vi "Main.vi"() -> ()   [LabVIEW 2015]
panel:
  out "data value":i32[][](array[numeric])
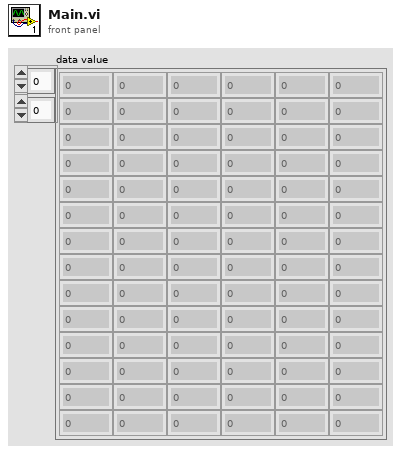
[diagram p1: front panel]
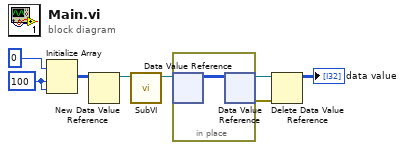
[diagram p0: block diagram]
diagram:
  w7 = 100 ("dimension size")
  n1 = Initialize Array(0, w7, w7) -> (w6:i32[][])
  n2 = New Data Value Reference(data value=w6) -> (data value reference=w5:refnum<data-value>)  [unwired: 1 in, 1 out]
  n3 = call "SubVI.vi"("Data Value Reference in"=w5) -> ("Data Value Reference out"=w4:refnum<data-value>)  [unwired: 10 in]
  n4 = in-place {
    n5 = in-place-dvr #1(w4) -> (w9:i32[][])  [unwired: 1 out]
    n6 = in-place-dvr #1(w9) -> (w3:refnum<data-value>, w1:errorcluster)
  }
  n7 = Delete Data Value Reference(data value reference=w3, error in=w1) -> (data value=→"data value":i32[][])  [unwired: 1 out]
